vi "(SubVI) Remove Threshold _YCC.vi"(4 "T=Larger\nF=Smaller":bool, 5 "Threshold":dbl, 6 "Ref":dbl[](array[numeric]), 7 "Signal":dbl[](array[numeric])) -> (3 "Signal Out":dbl[](array[numeric]))   [LabVIEW 2014]
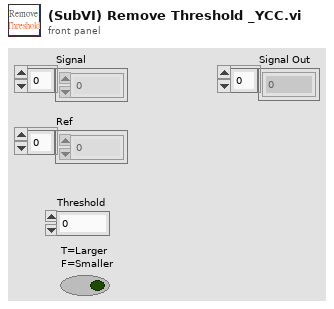
[diagram p1: front panel]
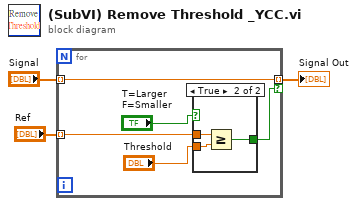
[diagram p0: block diagram]
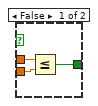
[diagram p2: hidden frame]
diagram:
  n1 = for {
    tunnel: "Signal" -> [w4] mode=indexing
    tunnel: [w4] -> w2 mode=indexing if=w6
    tunnel: "Ref" -> [w5] mode=indexing
    n2 = case shown="True" "T=Larger\nF=Smaller" {
      tunnel: "Threshold" -> [w11 w14]
      tunnel: [w10 w13] -> w6
      tunnel: w5 -> [w9 w12]
      frame False {
        n3 = Less Or Equal?(x=w9, y=w11) -> (x <= y?=w10:bool)
      }
      frame True {
        n4 = Greater Or Equal?(x=w12, y=w14) -> (x >= y?=w13:bool)
      }
    }
  }
  "Signal Out" <- w2
